vi "RemoveOutToFile.vi"(8 "ErrorArray In":errorcluster[](array[cluster])) -> (0 "ErrorArray Out":errorcluster[](array[cluster]))   [LabVIEW 2017, in "Bus_class.lvlib" / "Bus.lvclass"]
uses:
  Bus.lvclass
  <userlib>/NIST/ModuleAdminLib/ModuleAdmin/ModuleAdmin.lvclass
  Framework.lvlib
  <userlib>/NIST/NISTErrorLib/NISTErrorLib.lvlib
  Modules/OutputToFileModule/OutputToFileModule.lvlib
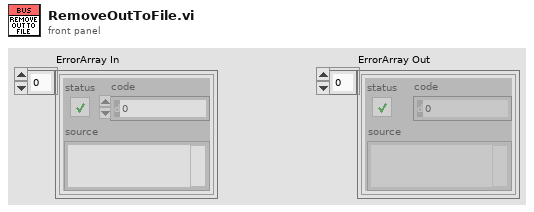
[diagram p1: front panel]
types:
  T1 = typedef "Framework.lvlib/clFrameworkData.ctl" = cluster{"EvtINIFilePaths":path[], "BusClassInstances":refnum<class "Bus.lvclass">[], "PmuImpairINIFilePaths":path[], "FlagImpairINIFilePaths":path[], "NetImpairINIFilePaths":path[], "OutputToFileINIFilePaths":path[], "AppINIFilePaths":path[], "AppModuleID":i32, "OutputToFileID":i32}
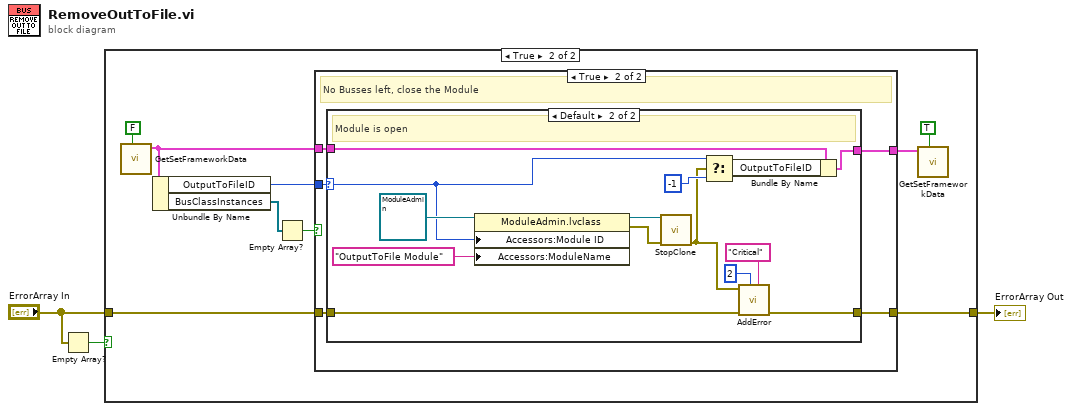
[diagram p0: block diagram]
diagram:
  n1 = Empty Array?(array="ErrorArray In") -> (empty?=w3:bool)
  n2 = case shown="True" w3 {
    tunnel: "ErrorArray In" -> [w4 w6]
    tunnel: [w4 w5] -> w1
    frame False {
    }
    frame True {
      n3 = call "GetSetFrameworkData.vi"("Set (F)"=FALSE) -> ("clFrameworkData Out"=w9:T1)  [unwired: 10 in]
      n4 = Unbundle By Name(w9) -> ("OutputToFileID"=w10:i32, "BusClassInstances"=w12:refnum<class "Bus.lvclass">[])
      n5 = Empty Array?(array=w12) -> (empty?=w11:bool)
      n6 = case shown="True" w11 {
        tunnel: w10 -> [_ w16]
        tunnel: w9 -> [w14 w20]
        tunnel: [w14 w19] -> w8
        tunnel: w6 -> [w15 w18]
        tunnel: [w15 w17] -> w5
        frame False {
          # "More Buses, Do nothing"
        }
        frame True {
          # "No Busses left, close the Module"
          n7 = case shown="Default" w16 {
            selector: w16 -> [_ w23]
            tunnel: w20 -> [w22 w32]
            tunnel: [w22 w31] -> w19
            tunnel: w18 -> [w21 w27]
            tunnel: [w21 w24] -> w17
            frame -1, 0 {
              # "App is not running"
            }
            frame Default {
              # "Module is open"
              n8 = property class="ModuleAdmin.lvclass"(reference=refnum<class "ModuleAdmin.lvclass"> refnum ("NistModuleAdmin.lvlib:NistModuleAdmin.lvclass"), "Accessors:Module ID"=w23, "Accessors:ModuleName"="OutputToFile Module" ("ModuleName")) -> (reference out=w34:refnum<class "ModuleAdmin.lvclass">, error out=w33:errorcluster)  [unwired: 1 in]
              n9 = call "StopClone.vi"("error in (no error)"=w33, "ModuleAdmin"=w34) -> ("error out"=w28:errorcluster)  [unwired: 9 in]
              n10 = Select(t=w23, s=w28, f=-1 ("AppModuleID")) -> (s? t:f=w30:i32)
              n11 = Bundle By Name(cluster=w32, "OutputToFileID"=w30) -> (w31:T1)
              n12 = call <userlib>:"AddError.vi"("Severity"="Critical", "Priority"=u8 2, "ErrorArray"=w27, "error in (no error)"=w28) -> ("ErrorArray"=w24:errorcluster[])  [unwired: 6 in, 1 out]
            }
          }
        }
      }
      n13 = call "GetSetFrameworkData.vi"("Set (F)"=TRUE, "clFrameworkData In"=w8) -> ()  [unwired: 9 in, 1 out]
    }
  }
  "ErrorArray Out" <- w1
